vi "fordmeplease.vi"() -> ()   [LabVIEW 2018]
panel:
  out "Test Points":dbl
  out "Test - Exam Answer Key":string
  out "Test - One Answer":string
  out "Test - All Answers":string
  out "Identification":string
  out "WHAT DO I SEE?":string
  out "Third Parse Output":string
  out "Second Parse Output":string
  out "First Parse Length":dbl
  out "First Parse Output":string
  out "Text Output":string
  in  "Path":path
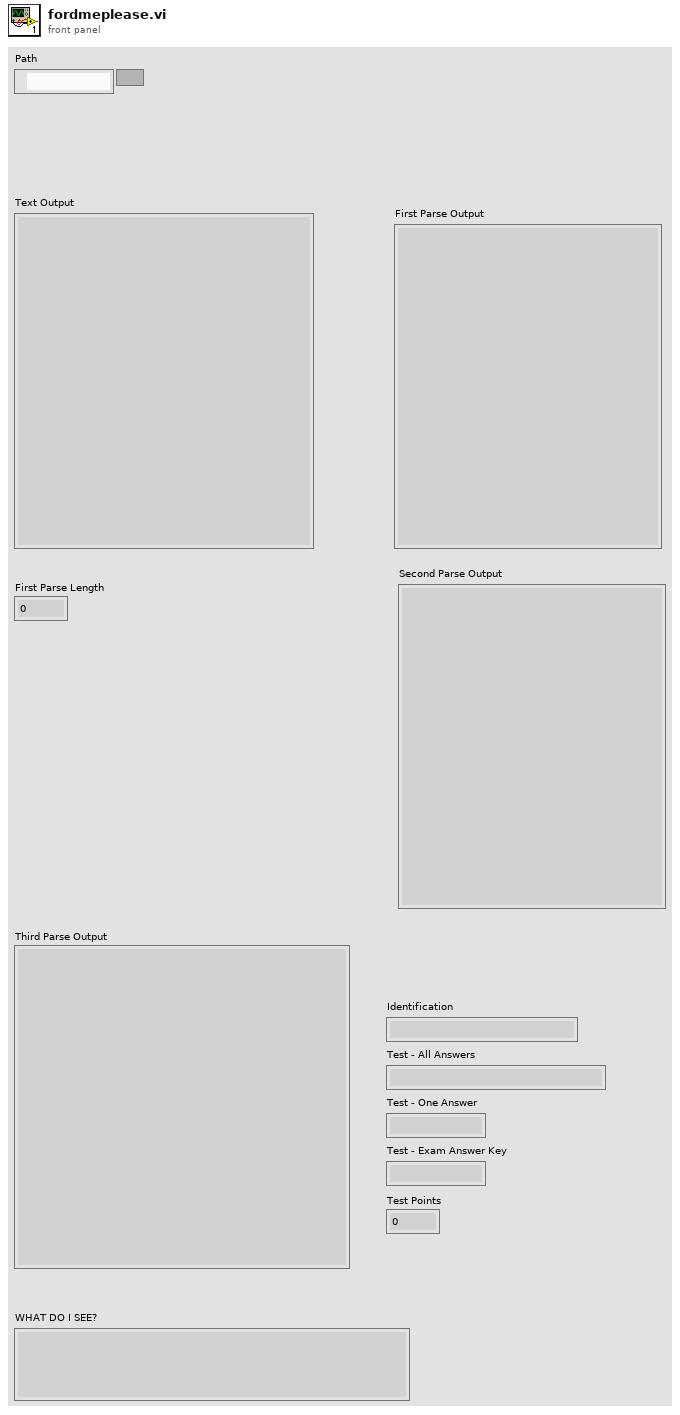
[diagram p1: front panel]
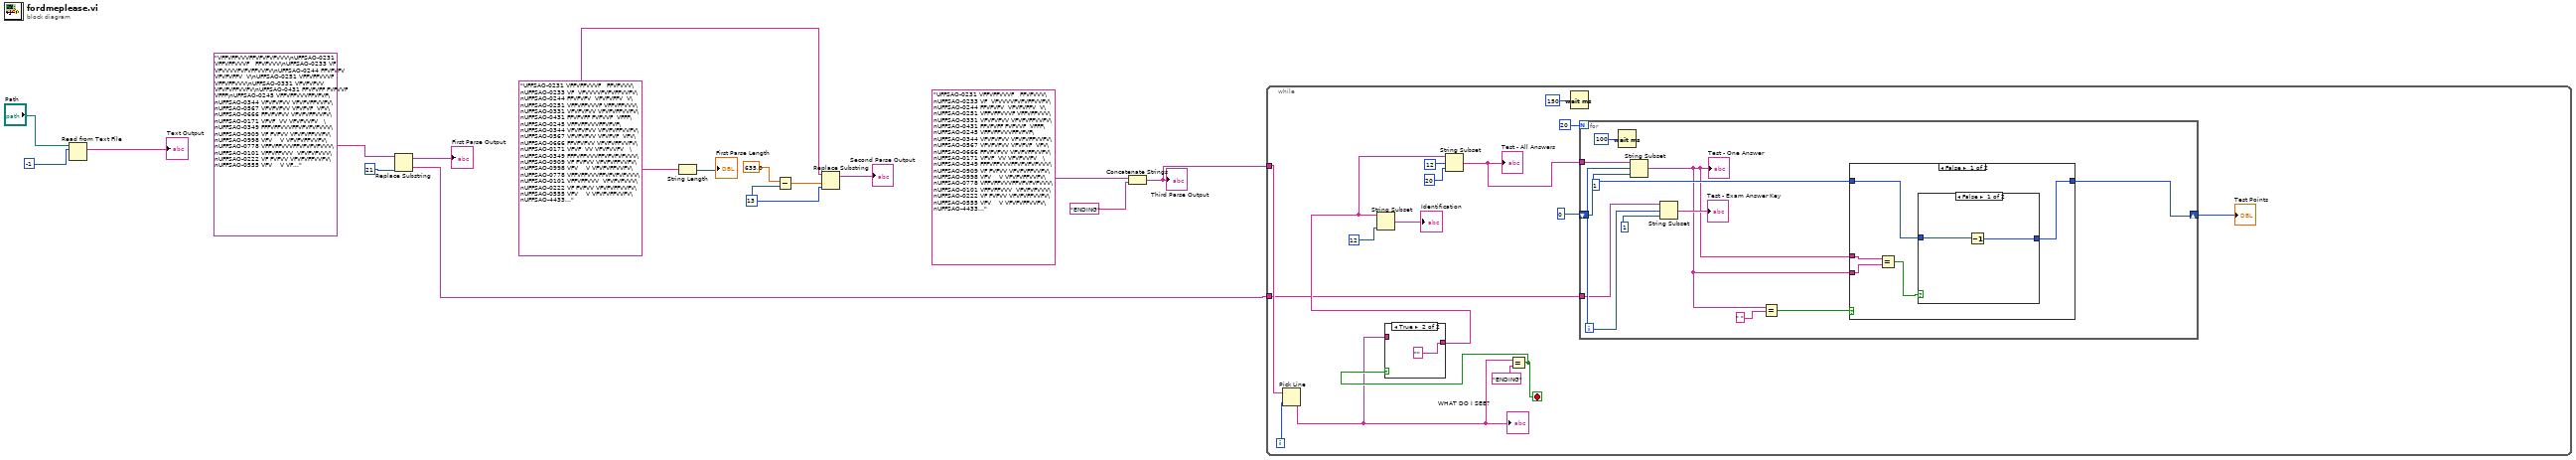
[diagram p0: block diagram]
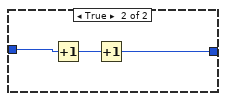
[diagram p2: hidden frame]
diagram:
  w9 = 13
  w8 = "UFFSAO-0231 VFFVFFVVVF   FFVFVVV\nUFFSAO-0233 VF  VFVVVVFVFVFFVVFV\nUFFSAO-0244 FFVFVFV  VFVFVFFV  V\nUFFSAO-0251 VFFVFFVVVF VFFVFFVVV\nUFFSAO-0331 VFVFVFVV VFVFVFFVVFV\nUFFSAO-0431 FFVFVFF FVFVVF  VFFF\nUFFSAO-0245 VFFVFFVVVFFVFVF\nUFFSAO-0344 VFVFVFVV VFVFVFFVVFV\nUFFSAO-0567 VFVFVFVV VFVFVF  VFV\nUFFSAO-0666 FFVFVFVV VFVFVFFVVFV\nUFFSAO-0171 VFVF  VV VFVFVVFV   \nUFFSAO-0349 FFFVFFVVVFFVFVFVFVVV\nUFFSAO-0909 VF FVFVV VFVFVFFVVFV\nUFFSAO-0998 VFV    V VFVFVFFVVFV\nUFFSAO-0778 VFFVFFVVVFFVFVFVFVVV\nUFFSAO-0101 VFFVFFVVV  VFVFVFVVV\nUFFSAO-0222 VF FVFVV VFVFVFFVVFV\nUFFSAO-0555 VFV    V VFVFVFFVVFV\nUFFSAO-4433 VFFVFFVVVFFVFVFVFVVV\nUFFSAO-0777  " ("Parsed Text Output")
  n1 = Read from Text File(file (use dialog)="Path", count=-1) -> (text=→"Text Output":string)  [unwired: 2 in, 3 out]
  n2 = Replace Substring(2:21, 5:"VFFVFFVVVFFVFVFVFVVV\nUFFSAO-0231 VFFVFFVVVF   FFVFVVV\nUFFSAO-0233 VF  VFVVVVFVFVFFVVFV\nUFFSAO-0244 FFVFVFV  VFVFVFFV  V\nUFFSAO-0251 VFFVFFVVVF VFFVFFVVV\nUFFSAO-0331 VFVFVFVV VFVFVFFVVFV\nUFFSAO-0431 FFVFVFF FVFVVF  VFFF\nUFFSAO-0245 VFFVFFVVVFFVFVF\nUFFSAO-0344 VFVFVFVV VFVFVFFVVFV\nUFFSAO-0567 VFVFVFVV VFVFVF  VFV\nUFFSAO-0666 FFVFVFVV VFVFVFFVVFV\nUFFSAO-0171 VFVF  VV VFVFVVFV   \nUFFSAO-0349 FFFVFFVVVFFVFVFVFVVV\nUFFSAO-0909 VF FVFVV VFVFVFFVVFV\nUFFSAO-0998 VFV    V VFVFVFFVVFV\nUFFSAO-0778 VFFVFFVVVFFVFVFVFVVV\nUFFSAO-0101 VFFVFFVVV  VFVFVFVVV\nUFFSAO-0222 VF FVFVV VFVFVFFVVFV\nUFFSAO-0555 VFV    V VFVFVFFVVFV\nUFFSAO-4433 VFFVFFVVVFFVFVFVFVVV\nUFFSAO-0777  " ("Text Output")) -> (0:w1:string, 1:→"First Parse Output":string)  [unwired: 2 in]
  n3 = String Length(string=w8) -> (length=→"First Parse Length":i32)
  n4 = Subtract(x=635.0 ("First Parse Length"), y=w9) -> (x-y=w10:dbl)
  n5 = Replace Substring(2:w9, 3:w10, 5:w8) -> (1:→"Second Parse Output":string)  [unwired: 1 in, 1 out]
  n6 = Concatenate Strings("UFFSAO-0231 VFFVFFVVVF   FFVFVVV\nUFFSAO-0233 VF  VFVVVVFVFVFFVVFV\nUFFSAO-0244 FFVFVFV  VFVFVFFV  V\nUFFSAO-0251 VFFVFFVVVF VFFVFFVVV\nUFFSAO-0331 VFVFVFVV VFVFVFFVVFV\nUFFSAO-0431 FFVFVFF FVFVVF  VFFF\nUFFSAO-0245 VFFVFFVVVFFVFVF\nUFFSAO-0344 VFVFVFVV VFVFVFFVVFV\nUFFSAO-0567 VFVFVFVV VFVFVF  VFV\nUFFSAO-0666 FFVFVFVV VFVFVFFVVFV\nUFFSAO-0171 VFVF  VV VFVFVVFV   \nUFFSAO-0349 FFFVFFVVVFFVFVFVFVVV\nUFFSAO-0909 VF FVFVV VFVFVFFVVFV\nUFFSAO-0998 VFV    V VFVFVFFVVFV\nUFFSAO-0778 VFFVFFVVVFFVFVFVFVVV\nUFFSAO-0101 VFFVFFVVV  VFVFVFVVV\nUFFSAO-0222 VF FVFVV VFVFVFFVVFV\nUFFSAO-0555 VFV    V VFVFVFFVVFV\nUFFSAO-4433 VFFVFFVVVFFVFVFVFVVV\n" ("First Parse Output 2"), "ENDING") -> (w2:string)
  "Third Parse Output" <- w2
  n7 = while {
    tunnel: w2 -> [w32]
    tunnel: w1 -> [w19]
    i -> [w31]
    stop <- w24 stop-if-true
    n8 = Pick Line(multi-line string=w32, line index=w31) -> (output string=w23:string)  [unwired: 1 in]
    "WHAT DO I SEE?" <- w23
    n9 = Equal?(x=w23, y="ENDING") -> (x = y?=w24:bool)
    n10 = case shown="True" w24 {
      tunnel: w23 -> [w56 _]
      tunnel: [w56 ""] -> w22
      frame False {
      }
      frame True {
      }
    }
    n11 = String Subset(string=w22, length (rest)=12) -> (substring=→"Identification":string)  [unwired: 1 in]
    n12 = String Subset(string=w22, offset (0)=12, length (rest)=20) -> (substring=w20:string)
    "Test - All Answers" <- w20
    n13 = Wait (ms)(milliseconds to wait=150) -> ()  [unwired: 1 out]
    n14 = for {
      N: 20 -> [_]
      tunnel: w20 -> [w44]
      tunnel: w19 -> [w39]
      shift-right: [w34] -> w17
      shift-left: 0 -> [w35]
      i -> [w40]
      n15 = Wait (ms)(milliseconds to wait=100) -> ()  [unwired: 1 out]
      n16 = String Subset(string=w44, offset (0)=w40, length (rest)=1) -> (substring=w33:string)
      "Test - One Answer" <- w33
      n17 = String Subset(string=w39, offset (0)=w40, length (rest)=1) -> (substring=→"Test - Exam Answer Key":string)
      n18 = Equal?(x=" ", y=w33) -> (x = y?=w36:bool)
      n19 = case shown="False" w36 {
        tunnel: w35 -> [w46 w55]
        tunnel: [w45 w55] -> w34
        tunnel: w33 -> [w49 _]
        tunnel: w33 -> [w48 _]
        frame False {
          n20 = Equal?(x=w49, y=w48) -> (x = y?=w47:bool)
          n21 = case shown="False" w47 {
            tunnel: w46 -> [w51 w53]
            tunnel: [w50 w52] -> w45
            frame False {
              n22 = Decrement(x=w51) -> (x-1=w50:i32)
            }
            frame True {
              n23 = Increment(x=w53) -> (x+1=w54:i32)
              n24 = Increment(x=w54) -> (x+1=w52:i32)
            }
          }
        }
        frame True {
        }
      }
    }
    "Test Points" <- w17
  }
